vi "Wavemeter Control.vi"() -> ()   [LabVIEW 2012]
uses:
  <vilib>/DAQmx/write.llb/DAQmx Write (Digital 1D Bool NChan 1Samp 1Line).vi
  <vilib>/DAQmx/miscellaneous.llb/DAQmx Fill In Error Info.vi
panel:
  in  "Switch to Wavemeter\n      Offline / Online\n           <--              -->":bool
  in  "stop":bool
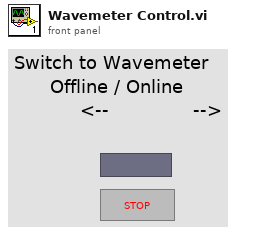
[diagram p1: front panel]
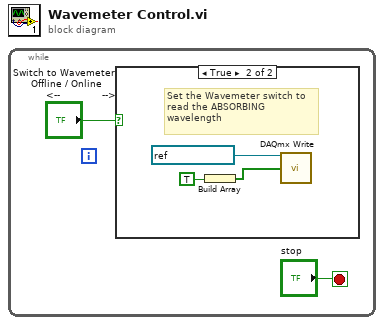
[diagram p0: block diagram]
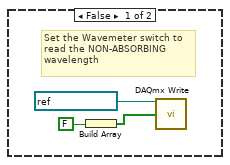
[diagram p2: hidden frame]
diagram:
  n1 = while {
    stop <- "stop" stop-if-true
    n2 = case shown="True" "Switch to Wavemeter\n      Offline / Online\n           <--              -->" {
      frame False {
        # "Set the Wavemeter switch to\nread the NON-ABSORBING\nwavelength"
        n3 = Build Array(FALSE ("Boolean")) -> (w3:bool[])
        n4 = call-poly <vilib>:"DAQmx Write.vi"("task/channels in"=refnum<k21> "BristolWM", "data"=w3) -> ()  [unwired: 11 in, 3 out]
      }
      frame True {
        # "Set the Wavemeter switch to\nread the ABSORBING\nwavelength"
        n5 = Build Array(TRUE ("Boolean")) -> (w6:bool[])
        n6 = call-poly <vilib>:"DAQmx Write.vi"("task/channels in"=refnum<k21> "BristolWM", "data"=w6) -> ()  [unwired: 11 in, 3 out]
      }
    }
  }
